vi "camara 3.vi"() -> ()   [LabVIEW 2010]
uses:
  <vilib>/addons/PixeLINK/Low Level Functions/CAMERA_FEATURES.llb/TDPU-CameraFeatures-PixelFormat.ctl
  <vilib>/sound2/lvsound2.llb/Sound Data Format.ctl
  <vilib>/sound2/lvsound2.llb/Sampling Mode.ctl
  <vilib>/Utility/error.llb/DialogType.ctl
  <vilib>/sound2/lvsound2.llb/Sound Output Task ID.ctl
  <vilib>/vision/Image Controls.llb/IMAQ Image.ctl
  <vilib>/addons/PixeLINK/Low Level Functions/ACQUISITION.llb/TDPU-Acquisition-StreamState.ctl
  <vilib>/addons/PixeLINK/Low Level Functions/CAMERA_FEATURES.llb/TDPU-CameraFeatures-FeatureFlags.ctl
  <vilib>/addons/PixeLINK/Low Level Functions/CAMERA_FEATURES.llb/TDPU-CameraFeatures-FeatureIds.ctl
  <vilib>/DAQmx/create/channels.llb/DAQmx Create Channel (AO-Voltage-Basic).vi
  <vilib>/DAQmx/configure/timing.llb/DAQmx Timing (Use Waveform).vi
panel:
  out "time elapsed (ms)":u32
  in  "Calibracion DAQ":T1
  in  "Secuencial":bool=TRUE
  in  "Freq Calibrador":dbl
  in  "Calibrar Sonido":bool
  out "Archivo Actual":path
  out "Guardando Imagen":bool=TRUE
  out "Freq Output":dbl
  out "Saltando":bool=TRUE
  out "Estable":bool=TRUE
  in  "Comienza Saltos":bool=TRUE
  in  "Nombre Imagen":string="foto"
  in  "Path":path
  in  "Parametros de Saltos":T2={"Numero de Saltos"=6, "Paso del Salto (Hz)"=100.0, "Tiempo de estabilizacion (s)"=1.0, "Frequencia de estabilizacion (Hz)"=2000.0, "Tiempo de rampa ON (s)"=5.0, "Tiempo de rampa OFF (s)"=1.0}
  in  "Numero Ultimo Experimento":i32
  in  "Tab Control":enum32{"Camara", "DAQ", "Control", "Sonido"}(tab)
  in  "Pixel Format Requerido":T3 items=["PIXEL_FORMAT_MONO8", "PIXEL_FORMAT_MONO16", "PIXEL_FORMAT_YUV422", "PIXEL_FORMAT_BAYER8_GRBG", "PIXEL_FORMAT_BAYER16_GRBG", "PIXEL_FORMAT_RGB24", "PIXEL_FORMAT_RGB48", "PIXEL_FORMAT_BAYER8_RGGB", "PIXEL_FORMAT_BAYER8_GBRG ", "PIXEL_FORMAT_BAYER8_BGGR ", "PIXEL_FORMAT_BAYER16_RGGB ", "PIXEL_FORMAT_BAYER16_GBRG", "PIXEL_FORMAT_BAYER16_BGGR", "PIXEL_FORMAT_RGB32"]
  in  "Exposure Time (ms)":dbl(slide) scale=0.1..2000.0
  in  "Gain":dbl(slide) scale=0.0..25.0
  in  "Red":sgl(slide) scale=0.0..4.0
  in  "Green":sgl(slide) scale=0.0..4.0
  in  "Blue":sgl(slide) scale=0.0..4.0
  in  "Selector":u16(ring) items=["776002034"]
  out "Numero de Camaras":u32
  in  "Camara ON?":bool
  in  "DAQ Parameters":T4={"Minimum Value"=-10.0, "Maximum Value"=10.0, "Physical Channel"="Dev1/ao0", "DAQ Fs (S/s)"=10000.0}
  in  "Ajuste ON?":bool
  in  "Control ON?":bool
  in  "Reset Control":bool
  in  "lamda (nm)":dbl=546.1
  in  "Control Parameters":T5={"N Init Avg"=6, "N Avg Best"=3, "% Best to test"=0.95, "% Best to beat"=1.0}
  in  "device ID":u32
  in  "sound format":T6={"sample rate (S/s)"=44000.0, "number of channels"=2, "bits per sample"=16}
  in  "Frecuencia":dbl(knob)=2000.0 scale=1000.0..4000.0
  in  "tiempo sonido (ms)":sgl=200.0
  out "Contraste":dbl(graph)
  out "Waveform":waveform(dbl)(graph)
  out "Image":T7(plugin-control)
  in  "Stop App":bool
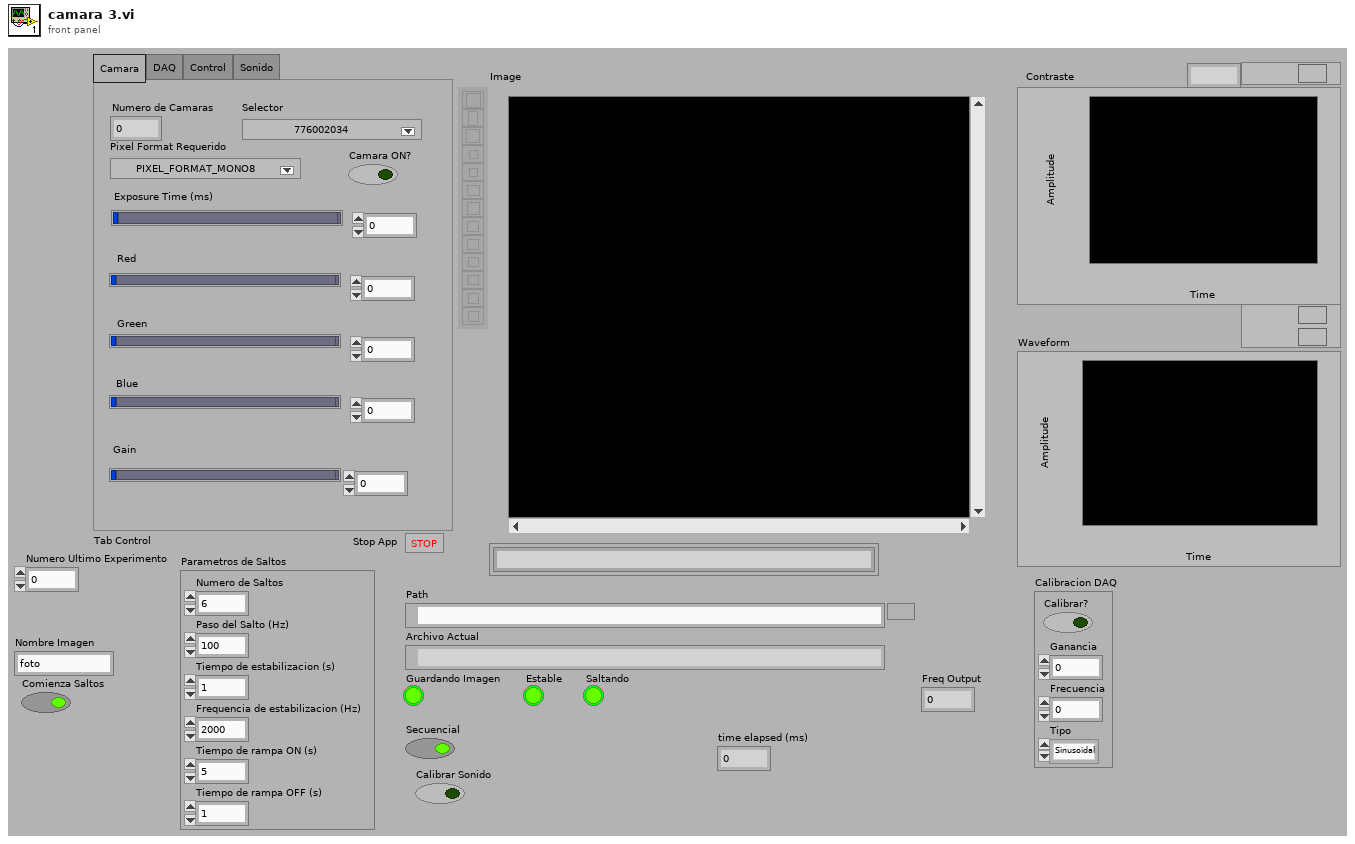
[diagram p1: front panel]
types:
  T1 = cluster{"Calibrar?":bool, "Ganancia":dbl, "Frecuencia":dbl, "Tipo":enum16{"Sinusoidal", "Triangular", "Cuadrada"}}
  T2 = cluster{"Numero de Saltos":i32, "Paso del Salto (Hz)":dbl, "Tiempo de estabilizacion (s)":dbl, "Frequencia de estabilizacion (Hz)":dbl, "Tiempo de rampa ON (s)":dbl, "Tiempo de rampa OFF (s)":dbl}
  T3 = typedef "TDPU-CameraFeatures-PixelFormat.ctl" = u16
  T4 = cluster{"Minimum Value":dbl, "Maximum Value":dbl, "Physical Channel":tag, "DAQ Fs (S/s)":dbl}
  T5 = cluster{"N Init Avg":u32, "N Avg Best":u32, "% Best to test":dbl, "% Best to beat":dbl}
  T6 = typedef "Sound Data Format.ctl" = cluster{"sample rate (S/s)":dbl, "number of channels":i32, "bits per sample":i32}
  T7 = typedef "IMAQ Image.ctl" = refnum<image>
  T8 = cluster{"time (ms)":dbl, "sound format":T6, "device ID":u32}
  T9 = cluster{"hCamera":u32, "Error":errorcluster, "uSerialNumber":u32}
  T10 = typedef "Sound Output Task ID.ctl" = u32
  T11 = cluster{"task ID":T10, "error":errorcluster, "sound format":T6}
  T12 = cluster{"DAQ Fs (S/s)":dbl, "task":refnum<k21>, "error":errorcluster, "Min Value":dbl, "Max Value":dbl}
  T13 = cluster{"Amplitud":dbl, "Media":dbl, "Sigma":dbl}
  T14 = typedef "DialogType.ctl" = u16
  T15 = typedef "Sampling Mode.ctl" = i32
  T16 = typedef "Image Type" = u32
  T17 = cluster{"sample rate (S/s)":dbl, "number of channels":i32, "bits per sample":i32}
  T18 = cluster{"hCamera":u32, "errorCamera":errorcluster}
  T19 = cluster{"hCamera":u32, "Error":errorcluster, "uSerialNumber OUT":u32}
  T20 = typedef "TDPU-Acquisition-StreamState.ctl" = u32
  T21 = typedef "TDPU-CameraFeatures-FeatureIds.ctl" = u32
  T22 = typedef "TDPU-CameraFeatures-FeatureFlags.ctl" = u32
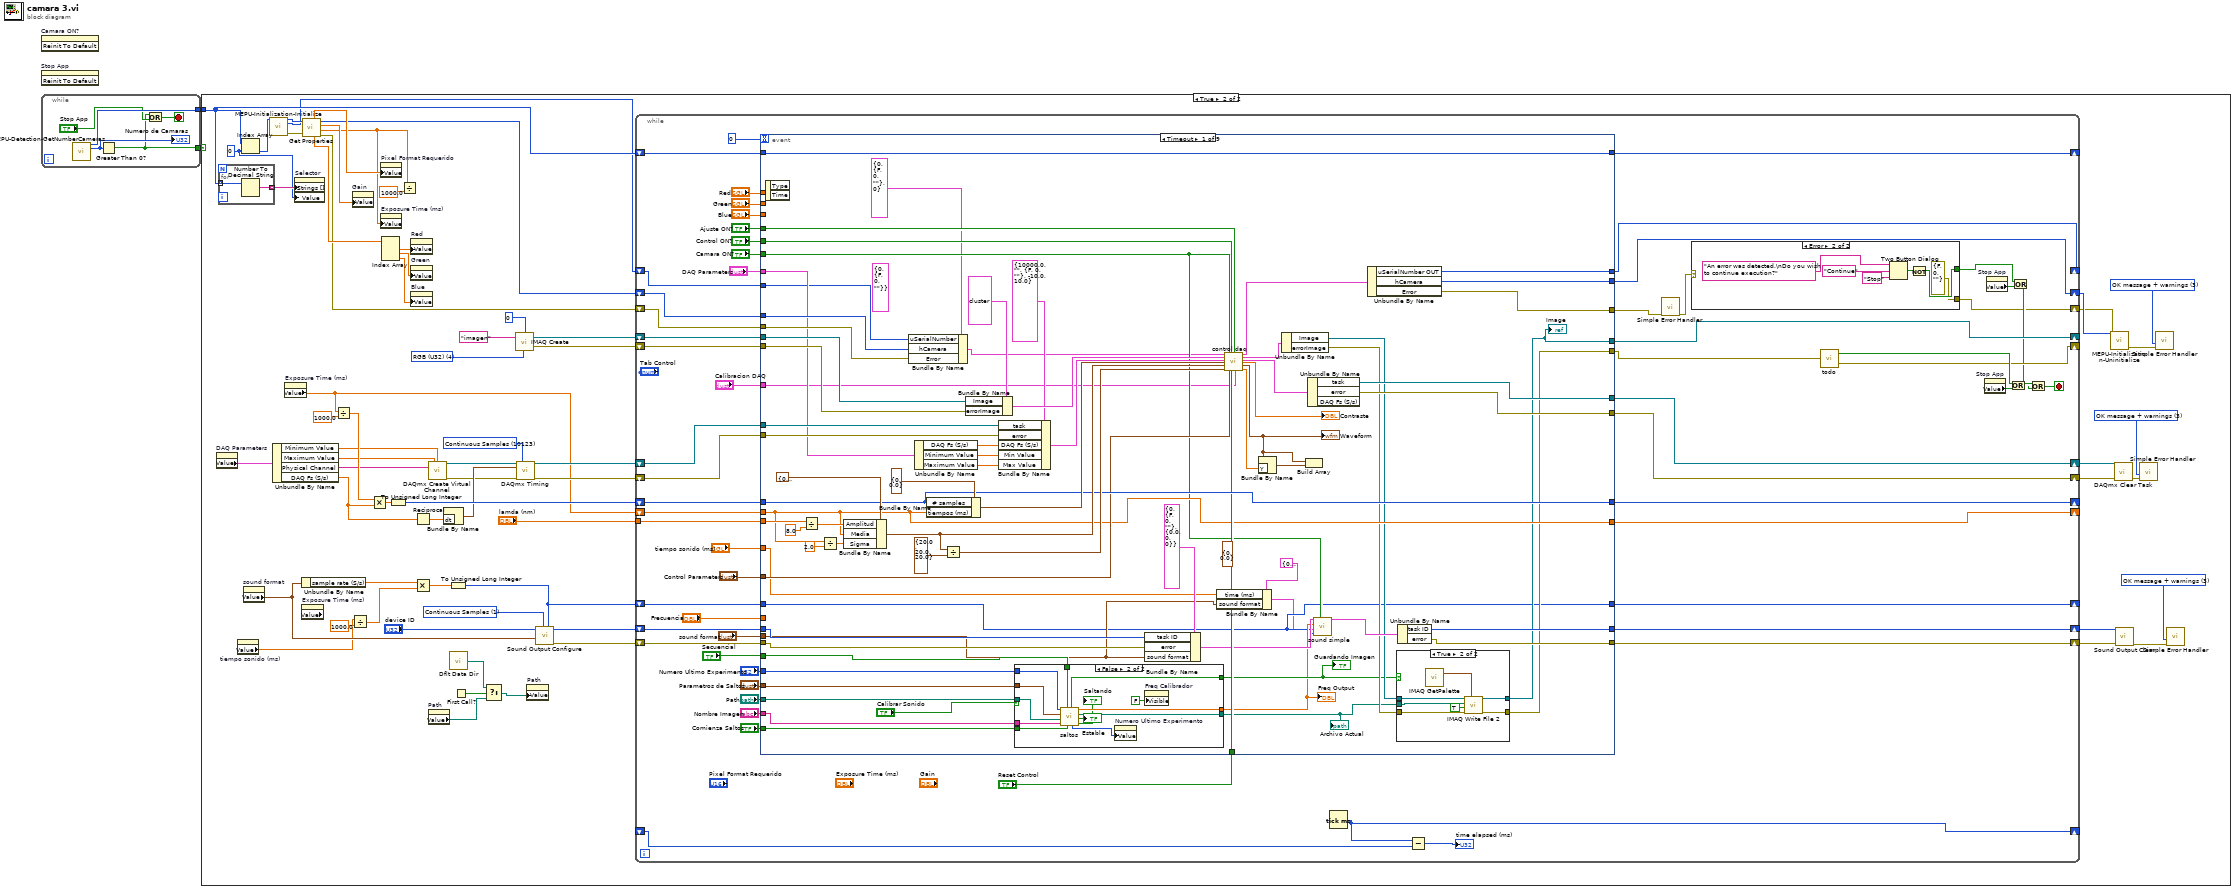
[diagram p0: block diagram]
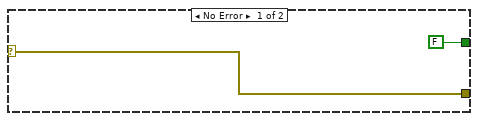
[diagram p3: hidden frame]
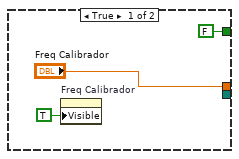
[diagram p4: hidden frame]
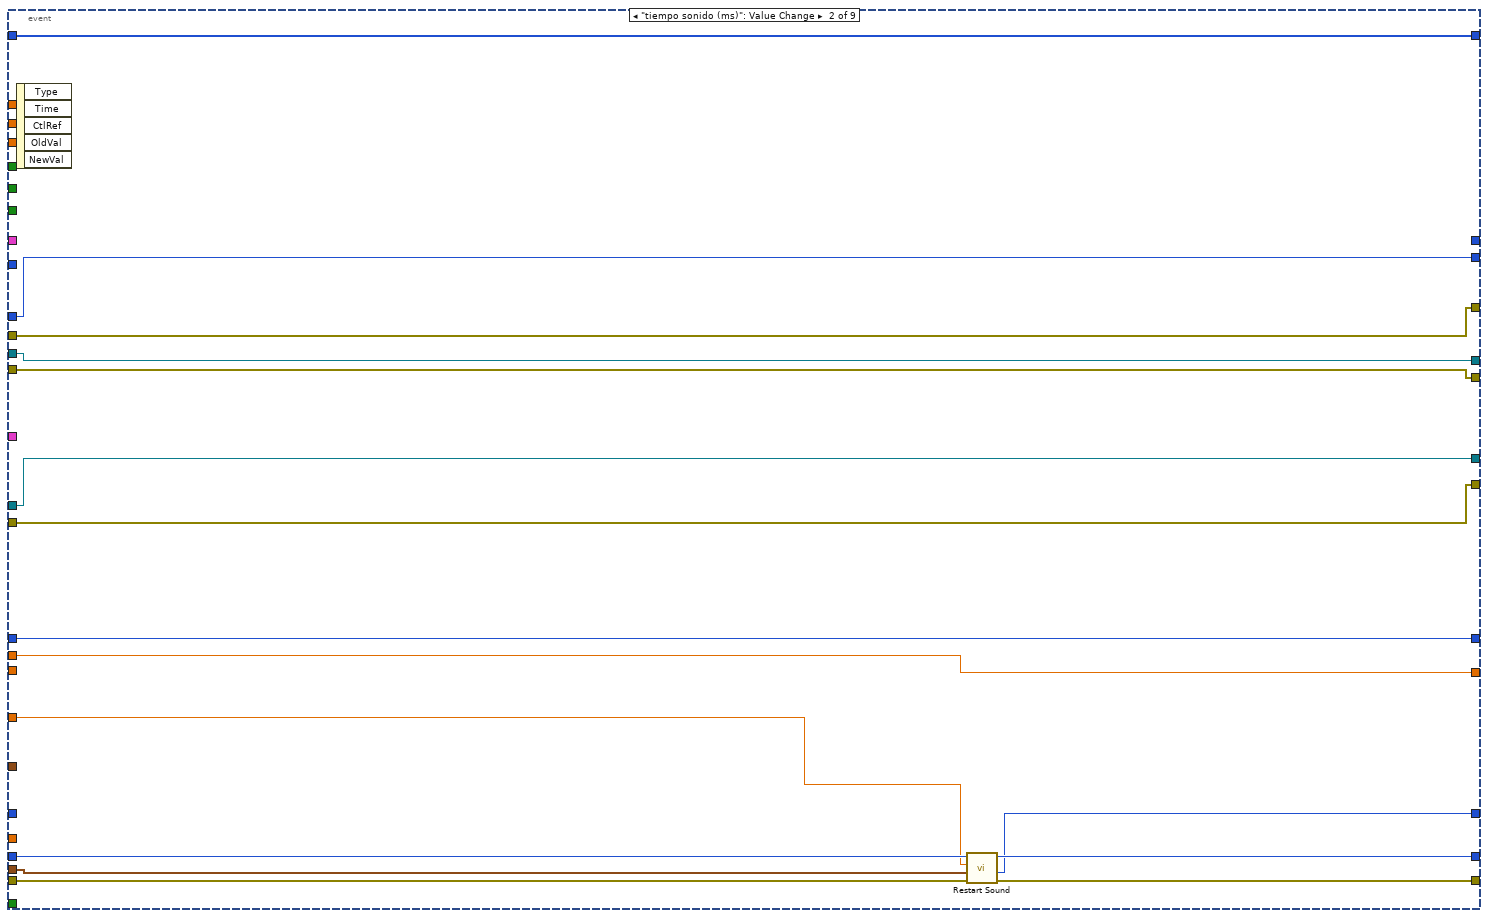
[diagram p6: hidden frame]
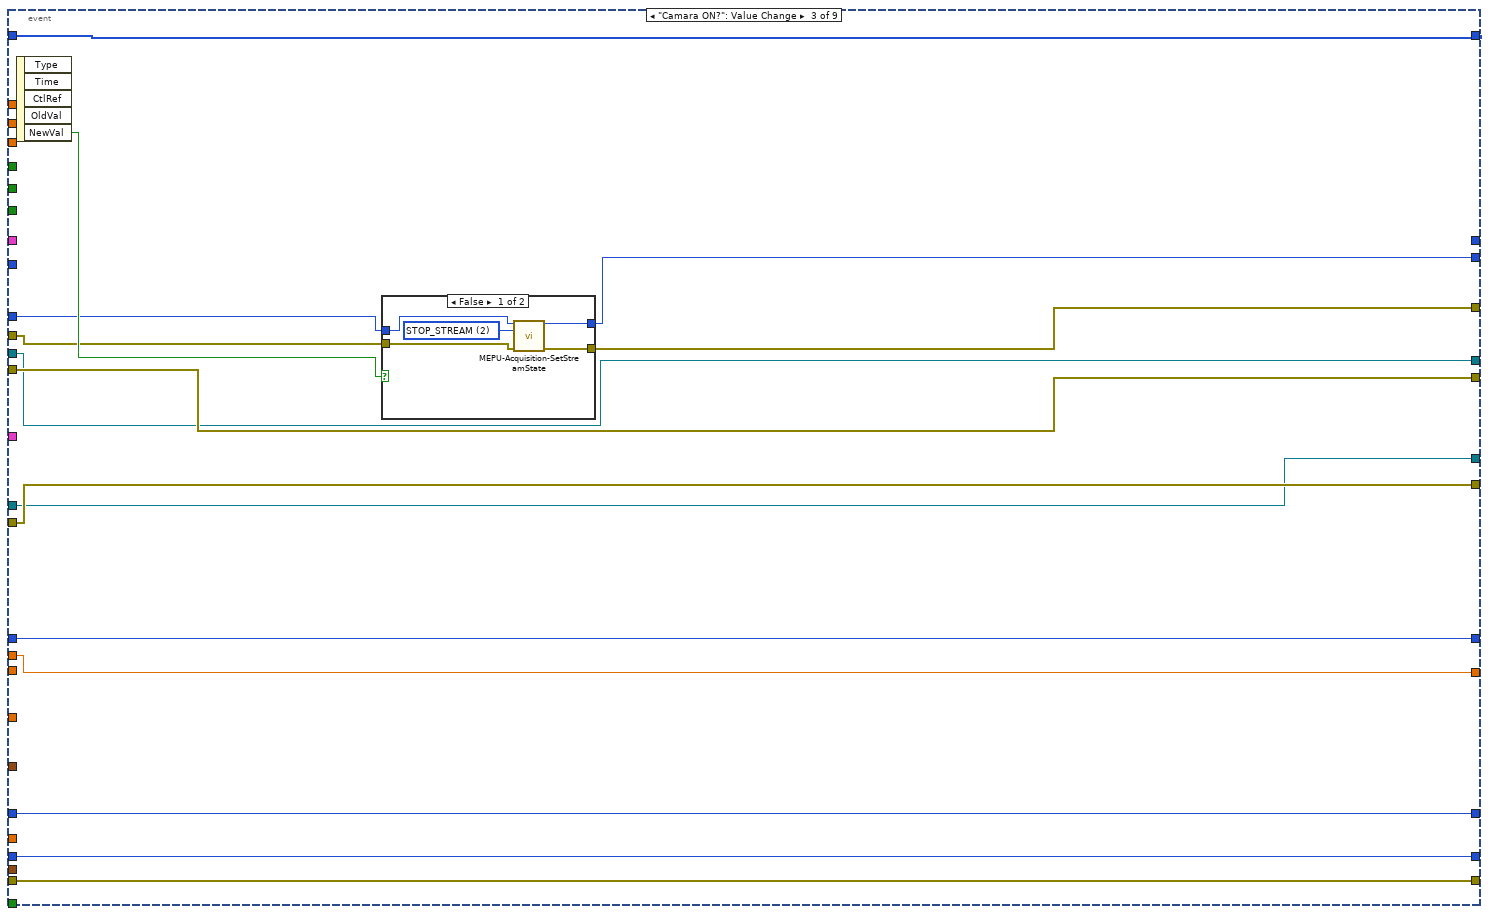
[diagram p7: hidden frame]
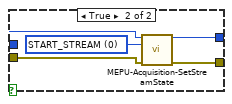
[diagram p8: hidden frame]
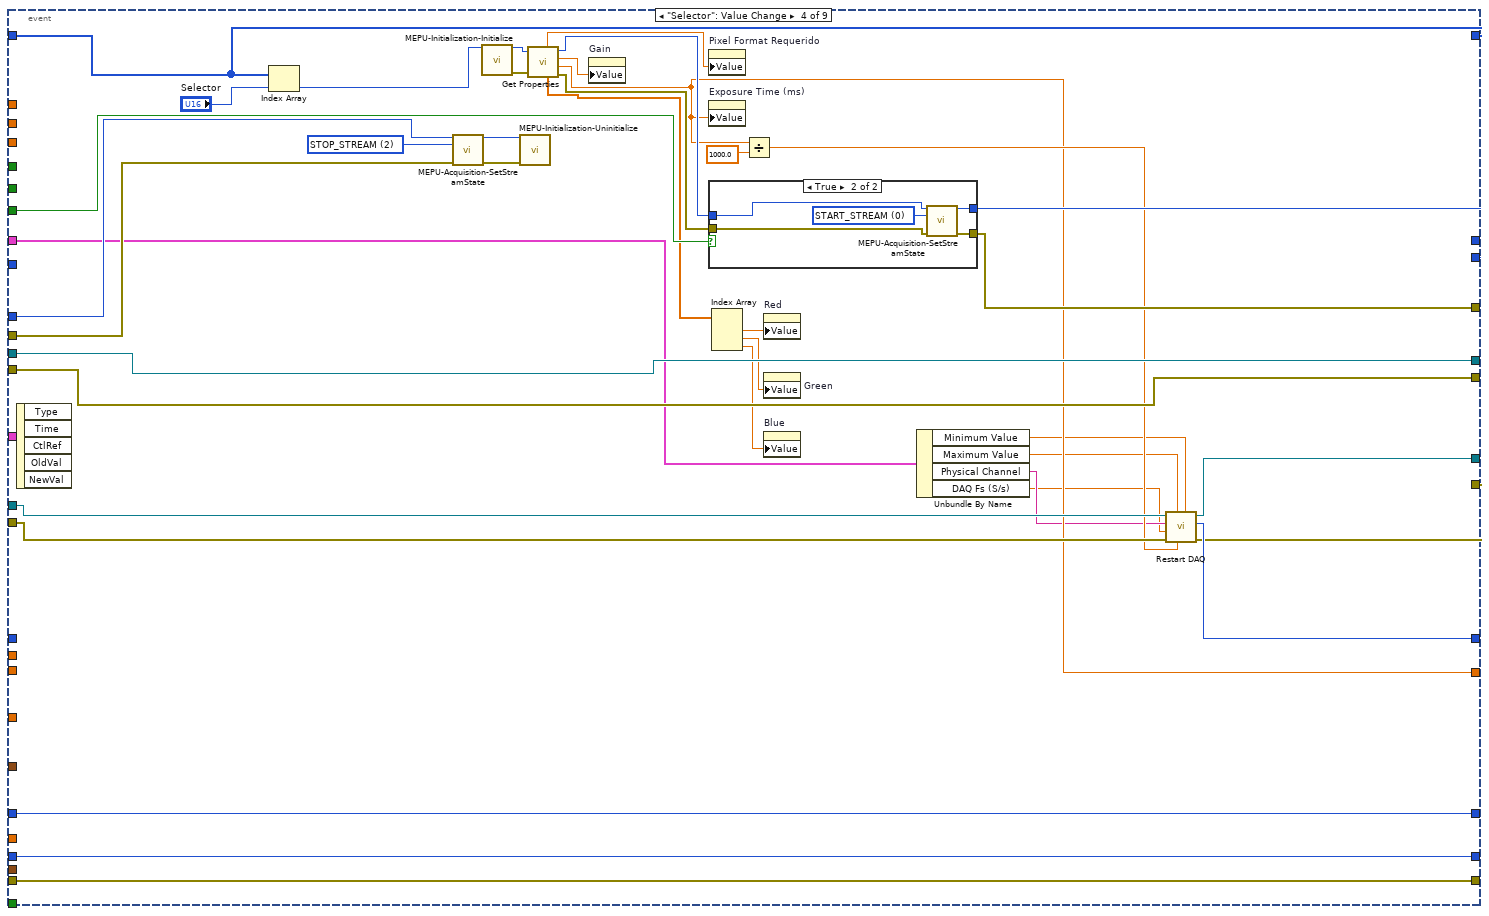
[diagram p9: hidden frame]
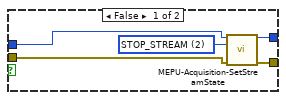
[diagram p10: hidden frame]
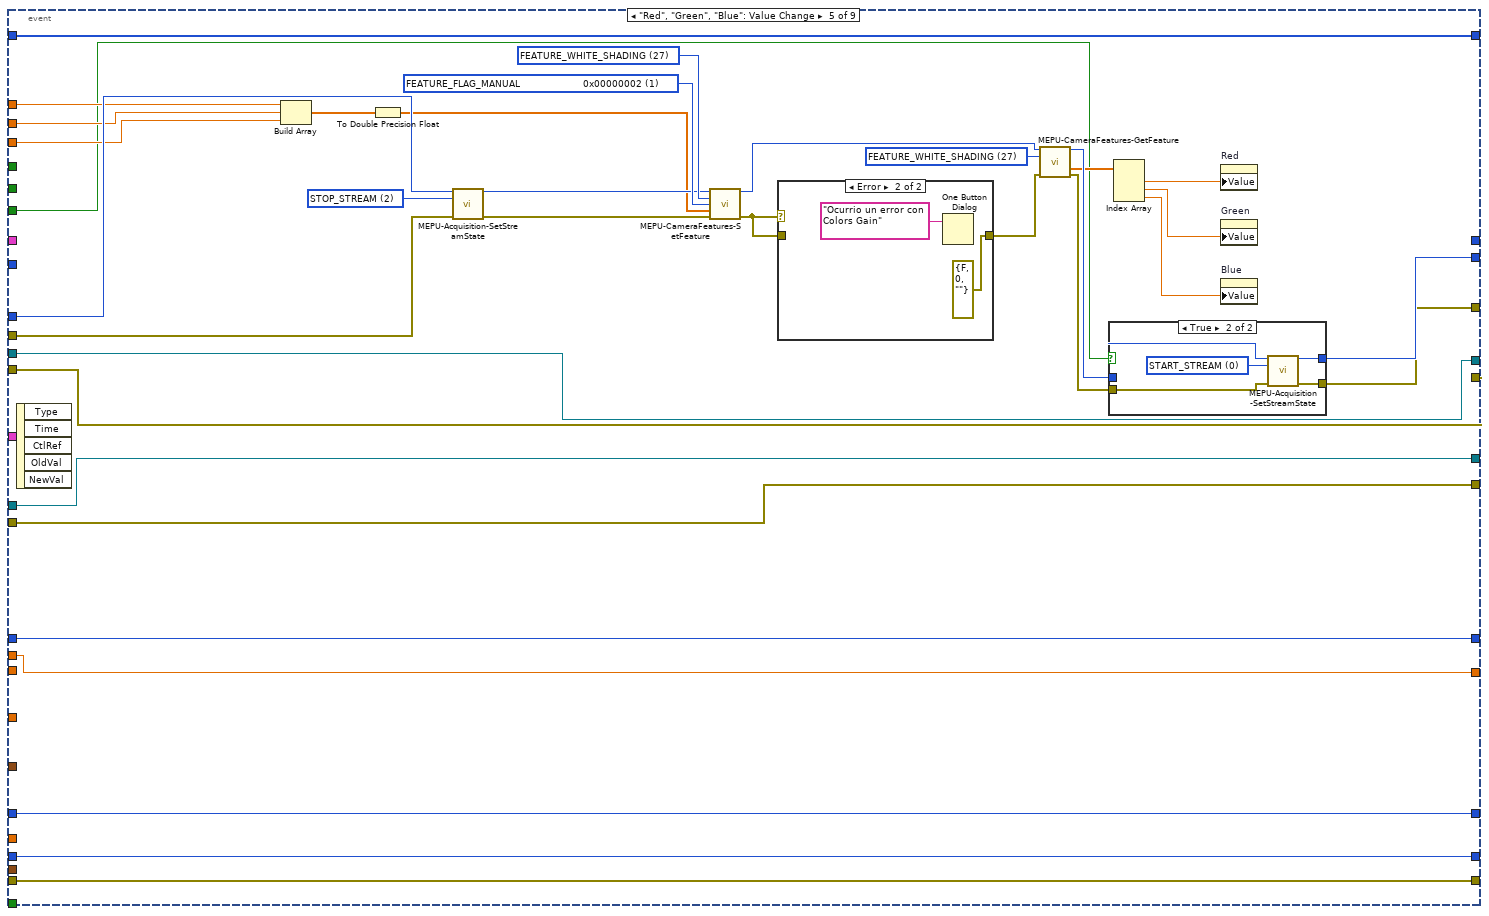
[diagram p11: hidden frame]
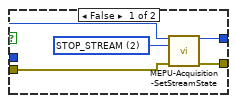
[diagram p12: hidden frame]
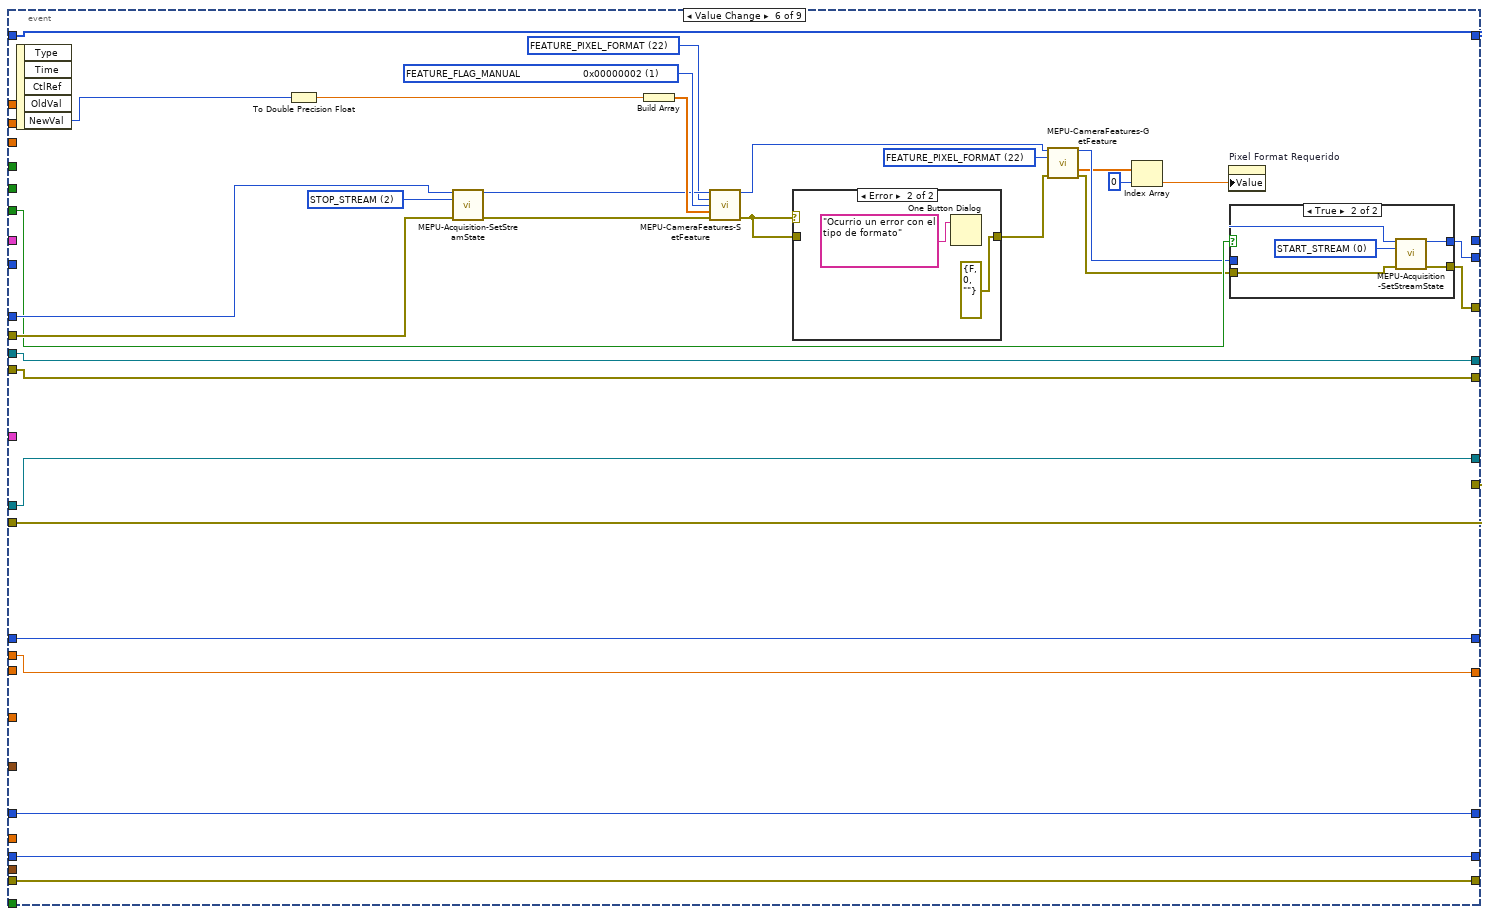
[diagram p14: hidden frame]
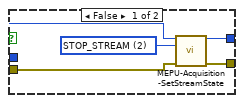
[diagram p15: hidden frame]
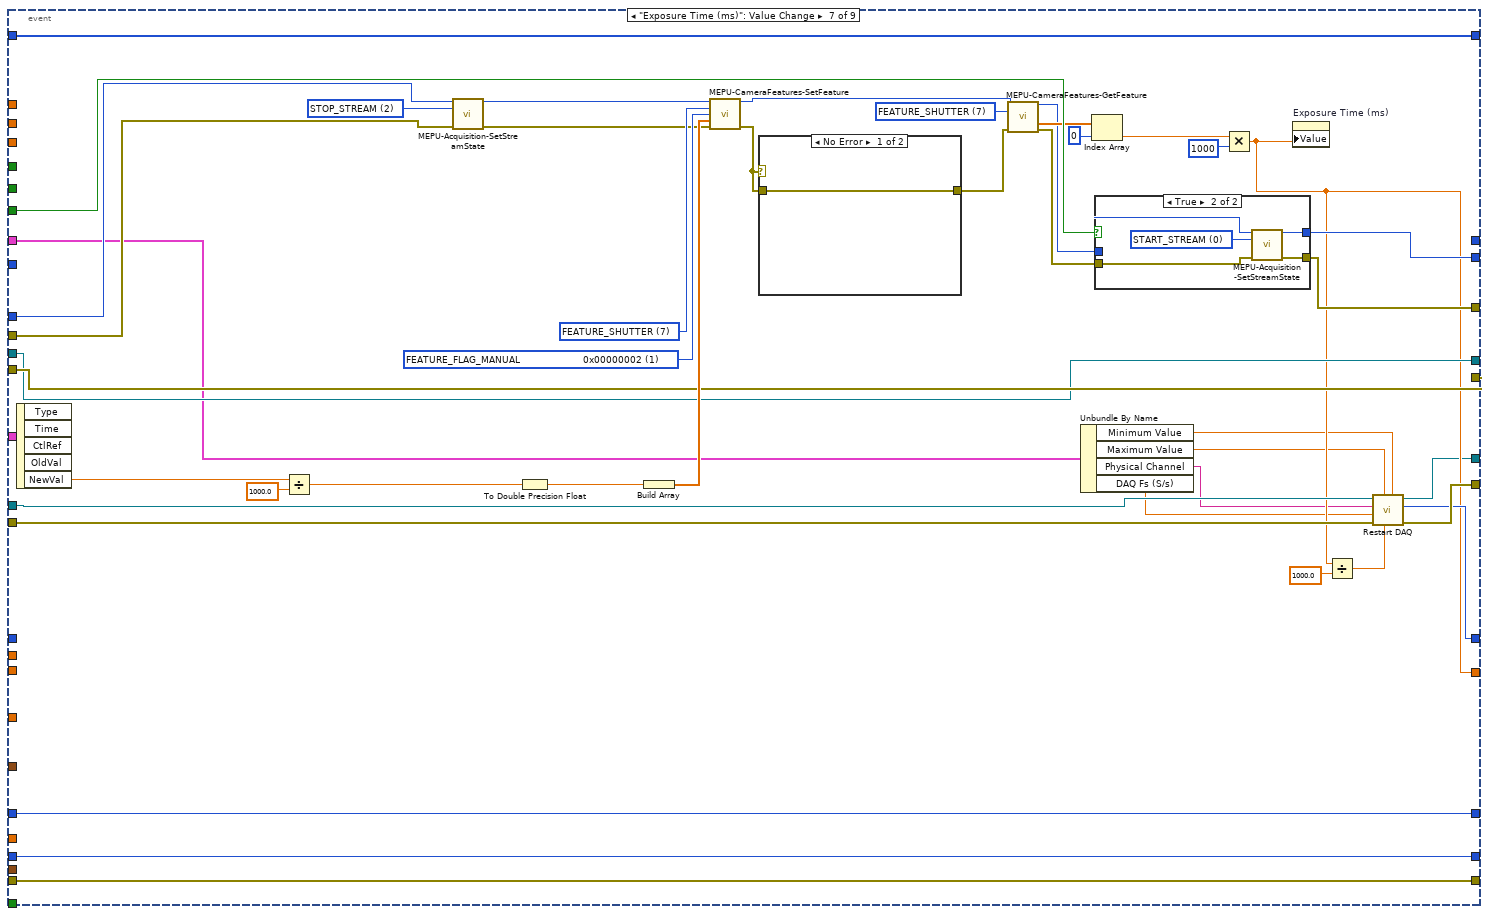
[diagram p17: hidden frame]
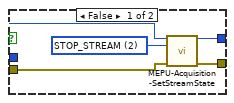
[diagram p18: hidden frame]
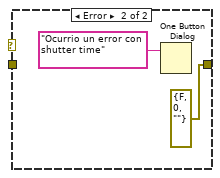
[diagram p19: hidden frame]
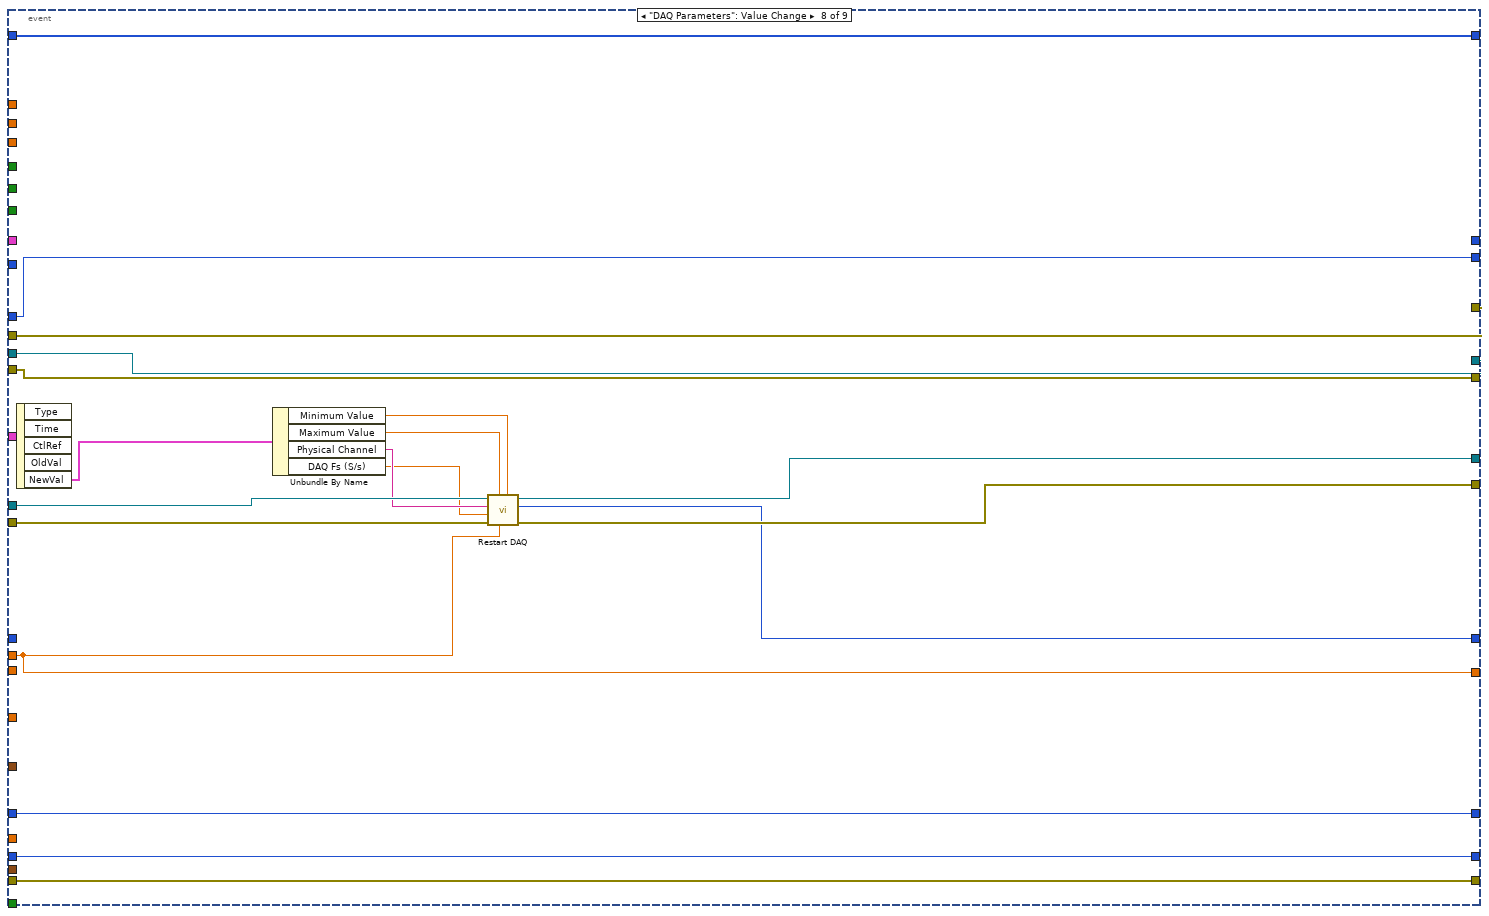
[diagram p20: hidden frame]
diagram:
  n1 = invoke on="Camara ON?" class="Bool (strict)" method="Reinit To Default"() -> ()  [unwired: 3 in, 3 out]
  n2 = invoke on="Stop App" class="Bool (strict)" method="Reinit To Default"() -> ()  [unwired: 3 in, 3 out]
  n3 = while {
    tunnel: [w7] -> w2
    tunnel: [w3] -> w1
    stop <- w5 stop-if-true
    n4 = call <vilib>:"MEPU-Detection-GetNumberCameras.vi"() -> ("LV_SerialNumbers OUT"=w7:u32[], "LV_NumberSerial OUT"=w4:u32)  [unwired: 13 in, 1 out]
    "Numero de Camaras" <- w4
    n5 = Greater Than 0?(x=w4) -> (x > 0?=w3:bool)
    n6 = Or(x=w3, y="Stop App") -> (x .or. y?=w5:bool)
  }
  n7 = case shown="True" w1 {
    tunnel: w2 -> [_ w72]
    frame False {
    }
    frame True {
      w23 = T14 3 items=["no dialog", "OK message", "continue or stop message", "OK message + warnings", "continue/stop + warnings"] ("type of dialog (OK msg:1)")
      w25 = T14 3 items=["no dialog", "OK message", "continue or stop message", "OK message + warnings", "continue/stop + warnings"] ("type of dialog (OK msg:1)")
      w35 = T15 1 items=["Finite Samples", "Continuous Samples"] ("sample mode")
      w38 = T14 3 items=["no dialog", "OK message", "continue or stop message", "OK message + warnings", "continue/stop + warnings"] ("type of dialog (OK msg:1)")
      w47 = 10123 items=["Finite Samples"=10178, "Continuous Samples"=10123, "Hardware Timed Single Point"=12522] ("sample mode")
      w66 = T16 4 items=["Grayscale (U8)", "Grayscale (I16)", "Grayscale (SGL)", "Complex (CSG)", "RGB (U32)", "HSL (U32)", "RGB (U64)", "Grayscale (U16)"] ("Image Type")
      w71 = 0
      n8 = property on="DAQ Parameters" class="Clust (strict)"() -> ("Value"=w16:T4)  [unwired: 2 in, 2 out]
      n9 = for {
        tunnel: w72 -> [w548] mode=indexing
        tunnel: [w547] -> w74 mode=indexing
        n10 = Number To Decimal String(number=w548) -> (decimal integer string=w547:string)  [unwired: 1 in]
      }
      n11 = property on="tiempo sonido (ms)" class="DigNum (strict)"() -> ("Value"=w14:sgl)  [unwired: 2 in, 2 out]
      n12 = Index Array(array=w72, index=w71) -> (element=w73:u32)
      n13 = property on="sound format" class="Clust (strict)"() -> ("Value"=w17:T17)  [unwired: 2 in, 2 out]
      n14 = call <vilib>:"MEPU-Initialization-Initialize.vi"("uSerialNumber IN"=w73) -> ("phCamera OUT"=w65:u32, "uSerialNumber OUT"=w9:u32, "Error OUT"=w64:errorcluster)  [unwired: 12 in]
      n15 = Unbundle By Name(w16) -> ("Minimum Value"=w20:dbl, "Maximum Value"=w19:dbl, "Physical Channel"=w15:tag, "DAQ Fs (S/s)"=w18:dbl)
      n16 = property on="Exposure Time (ms)" class="Slide (strict)"() -> ("Value"=w40:dbl)  [unwired: 2 in, 2 out]
      n17 = property on="Selector" class="Ring (strict)"("Strings []"=w74, "Value"=w71) -> ()  [unwired: 2 in, 2 out]
      n18 = Unbundle By Name(w17) -> ("sample rate (S/s)"=w31:dbl)
      n19 = property on="Exposure Time (ms)" class="Slide (strict)" props=["Value"]() -> ()  [unwired: 2 in, 3 out]
      n20 = call "Get Properties.vi"("hCamera IN"=w65, "Error IN"=w64) -> ("Pixel Format OUT"=w63:dbl, "hCamera OUT"=w49:u32, "Gain OUT"=w62:dbl, "Colors Gain OUT"=w58:dbl[], "Shutter Time OUT (ms)"=w55:dbl, "Error OUT"=w48:errorcluster)  [unwired: 3 in]
      n21 = Divide(x=w40, y=sgl 1000.0) -> (x/y=w51:dbl)
      n22 = Divide(x=w14, y=sgl 1000.0) -> (x/y=w30:sgl)
      n23 = property on="Gain" class="Slide (strict)"("Value"=w62) -> ()  [unwired: 2 in, 2 out]
      n24 = Multiply(x=w51, y=w18) -> (x*y=w57:dbl)
      n25 = property on="Pixel Format Requerido" class="Ring (strict)"("Value"=w63) -> ()  [unwired: 2 in, 2 out]
      n26 = property on="Exposure Time (ms)" class="Slide (strict)"("Value"=w55) -> ()  [unwired: 2 in, 2 out]
      n27 = Index Array(array=w58) -> (element #1=w61:dbl, element #2=w60:dbl, element #3=w59:dbl)  [unwired: 3 in]
      n28 = To Unsigned Long Integer(number=w57) -> (unsigned 32bit integer=w53:u32)
      n29 = Divide(x=w55, y=sgl 1000.0) -> ()  [unwired: 1 out]
      n30 = property on="Red" class="Slide (strict)"("Value"=w61) -> ()  [unwired: 2 in, 2 out]
      n31 = property on="Green" class="Slide (strict)"("Value"=w60) -> ()  [unwired: 2 in, 2 out]
      n32 = property on="Blue" class="Slide (strict)"("Value"=w59) -> ()  [unwired: 2 in, 2 out]
      n33 = Reciprocal(x=w18) -> (1/x=w45:dbl)
      n34 = Multiply(x=w31, y=w30) -> (x*y=w34:dbl)
      n35 = call-poly <vilib>:"DAQmx Create Virtual Channel.vi"("maximum value"=w19, "minimum value"=w20, "physical channels"=w15) -> ("task out"=w44:refnum<k21>, "error out"=w43:errorcluster)  [unwired: 11 in]
      n36 = property on="Path" class="Path"() -> ("Value"=w11:path)  [unwired: 2 in, 2 out]
      n37 = Bundle By Name("dt"=w45) -> (w46:waveform(dbl))  [unwired: 1 in]
      n38 = To Unsigned Long Integer(number=w34) -> (unsigned 32bit integer=w21:u32)
      n39 = call <vilib>:"Dflt Data Dir.vi"() -> ("App:Default Data Directory"=w10:path)
      n40 = First Call?() -> (First Call?: T/F=w13:bool)
      n41 = Select(t=w10, s=w13, f=w11) -> (s? t:f=w12:path)
      n42 = call "IMAQ Create"("Border Size"=0, "Image Name"="imagen", "Image Type"=w66) -> ("New Image"=w69:T7, "error out"=w67:errorcluster)  [unwired: 2 in]
      n43 = call-poly <vilib>:"DAQmx Timing.vi"("task/channels in"=w44, "sample mode"=w47, "waveform"=w46, "error in"=w43) -> ("task out"=w42:refnum<k21>, "error out"=w41:errorcluster)  [unwired: 10 in]
      n44 = property on="Path" class="Path"("Value"=w12) -> ()  [unwired: 2 in, 2 out]
      n45 = call <vilib>:"Sound Output Configure.vi"("number of samples/ch"=w21, "sample mode"=w35, "sound format"=w17, "device ID"="device ID") -> ("error out"=w29:errorcluster, "task ID"=w28:T10)  [unwired: 6 in]
      n46 = while {
        shift-right: [w133] -> _
        shift-left: w72 -> [w134]
        shift-right: [w107] -> w70
        shift-left: w49 -> [w132]
        shift-right: [w106] -> w54
        shift-left: w48 -> [w131]
        shift-right: [w113] -> _
        shift-left: w67 -> [w119]
        shift-right: [w118] -> _
        shift-left: w69 -> [w124]
        shift-right: [w114] -> _
        shift-left: w40 -> [w109]
        tunnel: "lamda (nm)" -> [w108]
        shift-right: [w103] -> _
        shift-left: w53 -> [w112]
        shift-right: [w99] -> w37
        shift-left: w42 -> [w101]
        shift-right: [w98] -> w36
        shift-left: w41 -> [w100]
        shift-right: [w94] -> w27
        shift-left: w28 -> [w96]
        shift-right: [w95] -> w26
        shift-left: w29 -> [w97]
        shift-right: [w92] -> _
        shift-left: w21 -> [w93]
        shift-right: [w79] -> _
        shift-left: w9 -> [w78]
        shift-right: [w76] -> _
        shift-left: _ -> [w77]
        stop <- w121 stop-if-true
        n47 = event shown="[0] Timeout" {
          selector: _ -> [_ _ _ _ _ _ _ _ _]
          dyn-events: _ -> [_ _ _ _ _ _ _ _ _]
          timeout: 0 -> [_ _ _ _ _ _ _ _ _]
          tunnel: w134 -> [w217 w258 w270 w320 w367 w404 w461 w501 w525]
          tunnel: [w196 w246 w268 w313 w351 w403 w460 w497 w524] -> w107
          tunnel: [w195 w247 w267 w314 w350 w402 w459 w498 w523] -> w126
          tunnel: [w217 w258 w270 w320 w367 w404 w461 w501 w525] -> w133
          tunnel: w132 -> [w216 w246 w266 w315 w353 w409 w458 w497 w522]
          tunnel: w131 -> [w215 w247 w265 w316 w352 w408 w457 w498 w521]
          tunnel: "Camara ON?" -> [w154 _ _ w312 w340 w401 w456 _ w520]
          tunnel: w124 -> [w212 w248 w271 w310 w355 w389 w442 w499 w511]
          tunnel: w119 -> [w211 w249 w272 w311 w354 w400 w453 w500 w519]
          tunnel: [w158 w249 w272 w311 w354 w400 w453 w500 w519] -> w123
          tunnel: [w160 w248 w271 w310 w355 w389 w442 w499 w511] -> w118
          tunnel: "Red" -> [_ _ _ _ w345 _ _ _ _]
          tunnel: "Green" -> [_ _ _ _ w344 _ _ _ _]
          tunnel: "Blue" -> [_ _ _ _ w343 _ _ _ _]
          tunnel: [w192 w250 w262 w296 w337 w384 w434 w494 w506] -> w99
          tunnel: [w191 w251 w263 w297 w336 w385 w440 w492 w505] -> w98
          tunnel: w109 -> [w178 w245 w269 _ w339 w387 _ w493 w508]
          tunnel: [w178 w245 w269 w292 w339 w387 w435 w493 w508] -> w114
          tunnel: w112 -> [w189 w252 w264 _ w338 w386 _ _ w507]
          tunnel: w108 -> [w198 _ _ _ _ _ _ _ _]
          tunnel: "Control ON?" -> [w210 _ _ _ _ _ _ _ _]
          tunnel: "Ajuste ON?" -> [w209 _ _ _ _ _ _ _ _]
          tunnel: [w189 w252 w264 w298 w338 w386 w439 w491 w507] -> w103
          tunnel: "Reset Control" -> [w188 _ _ _ _ _ _ _ _]
          tunnel: w101 -> [w186 w250 w262 w295 w337 w384 w438 w496 w506]
          tunnel: w100 -> [w185 w251 w263 w294 w336 w385 w437 w495 w505]
          tunnel: w97 -> [w181 w255 w261 w284 w333 w381 w428 w488 w503]
          tunnel: w96 -> [w182 w254 w260 w285 w334 w382 w426 w489 w502]
          tunnel: [w175 w257 w261 w284 w333 w381 w428 w488 w503] -> w95
          tunnel: [w176 w256 w260 w285 w334 w382 w426 w489 w502] -> w94
          tunnel: w93 -> [w144 _ w259 w286 w335 w383 w427 w490 w504]
          tunnel: "sound format" -> [w145 w243 _ _ _ _ _ _ _]
          tunnel: "Control Parameters" -> [w179 _ _ _ _ _ _ _ _]
          tunnel: "Frecuencia" -> [_ _ _ _ _ _ _ _ _]
          tunnel: [w144 w253 w259 w286 w335 w383 w427 w490 w504] -> w92
          tunnel: "DAQ Parameters" -> [w171 _ _ w291 _ _ w429 _ _]
          tunnel: "tiempo sonido (ms)" -> [w167 w244 _ _ _ _ _ _ _]
          tunnel: "Numero Ultimo Experimento" -> [w166 _ _ _ _ _ _ _ _]
          tunnel: "Parametros de Saltos" -> [w165 _ _ _ _ _ _ _ _]
          tunnel: "Path" -> [w164 _ _ _ _ _ _ _ _]
          tunnel: "Nombre Imagen" -> [w163 _ _ _ _ _ _ _ _]
          tunnel: "Comienza Saltos" -> [w162 _ _ _ _ _ _ _ _]
          tunnel: "Secuencial" -> [w152 _ _ _ _ _ _ _ _]
          tunnel: "Calibracion DAQ" -> [w151 _ _ _ _ _ _ _ _]
          tunnel: w78 -> [w148 _ _ _ _ _ _ _ _]
          tunnel: [w147 _ _ _ _ _ _ _ _] -> w79
          event Timeout {
            (unwired) cluster{"# samples":u32, "tiempos (ms)":dbl} {"# samples"=0, "tiempos (ms)"=0.0} ("Sound Parameters")
            (unwired) T18 {"hCamera"=0, "errorCamera"={"status"=FALSE, "code"=0, "source"=""}} ("Camera Device IN")
            n48 = event-data() -> ()  [unwired: 1 in, 2 out]
            n49 = Divide(x=w198, y=8.0) -> (x/y=w202:dbl)
            n50 = Divide(x=w178, y=2.0) -> (x/y=w205:dbl)
            n51 = Bundle By Name(cluster=T13 {"Amplitud"=0.0, "Media"=0.0, "Sigma"=0.0} ("Parametros Maximos"), "Amplitud"=w202, "Media"=w178, "Sigma"=w205) -> (w200:T13)
            n52 = Bundle By Name(cluster=T9 {"hCamera"=0, "Error"={"status"=FALSE, "code"=0, "source"=""}, "uSerialNumber"=0} ("Camera Device  IN"), "uSerialNumber"=w148, "hCamera"=w216, "Error"=w215) -> (w149:T9)
            n53 = Unbundle By Name(w171) -> ("DAQ Fs (S/s)"=w174:dbl, "Minimum Value"=w173:dbl, "Maximum Value"=w172:dbl)
            n54 = Bundle By Name(cluster=cluster{"# samples":u32, "tiempos (ms)":dbl} {"# samples"=0, "tiempos (ms)"=0.0} ("Sound Parameters"), "# samples"=w189, "tiempos (ms)"=w178) -> (w207:cluster{"# samples":u32, "tiempos (ms)":dbl})
            n55 = Divide(x=w200, y=T13 {"Amplitud"=20.0, "Media"=20.0, "Sigma"=20.0}) -> (x/y=w199:T13)
            n56 = Bundle By Name(cluster=cluster{"Image":T7, "errorImage":errorcluster} {"Image"=refnum, "errorImage"={"status"=FALSE, "code"=0, "source"=""}} ("Image Device IN"), "Image"=w212, "errorImage"=w211) -> (w213:cluster{"Image":T7, "errorImage":errorcluster})
            n57 = Bundle By Name(cluster=T12 {"DAQ Fs (S/s)"=10000.0, "task"="", "error"={"status"=FALSE, "code"=0, "source"=""}, "Min Value"=-10.0, "Max Value"=10.0} ("DAQ Device"), "task"=w186, "error"=w185, "DAQ Fs (S/s)"=w174, "Min Value"=w173, "Max Value"=w172) -> (w187:T12)
            n58 = case shown="False" "Calibrar Sonido" {
              tunnel: w166 -> [_ w233]
              tunnel: w165 -> [_ w232]
              tunnel: w164 -> [_ w231]
              tunnel: w163 -> [_ w230]
              tunnel: w162 -> [_ w229]
              tunnel: [_ w228] -> w157
              tunnel: [FALSE ("Captura Imagen") w227] -> w156
              tunnel: ["Freq Calibrador" w226] -> w155
              tunnel: w152 -> [_ w221]
              frame True {
                n59 = property on="Freq Calibrador" class="DigNum (strict)"("Visible"=TRUE) -> ()  [unwired: 2 in, 2 out]
              }
              frame False {
                n60 = call "saltos.vi"("Comienza Saltos"=w229, "Secuencial"=w221, "Nombre Imagen"=w230, "Path"=w231, "Parametros de Saltos"=w232, "Numero Ultimo Experimento"=w233) -> ("Tomando Saltos"=→"Saltando":bool, "Estable"=→"Estable":bool, "appended path"=w228:path, "Freq Output"=w226:dbl, "Numero Actual Experimento"=w225:i32, "Captura Imagen"=w227:bool)
                n61 = property on="Numero Ultimo Experimento" class="DigNum (strict)"("Value"=w225) -> ()  [unwired: 2 in, 2 out]
                n62 = property on="Freq Calibrador" class="DigNum (strict)"("Visible"=FALSE) -> ()  [unwired: 2 in, 2 out]
              }
            }
            "Freq Output" <- w155
            "Guardando Imagen" <- w156
            "Archivo Actual" <- w157
            n63 = Bundle By Name(cluster=T11 {"task ID"=0, "error"={"status"=FALSE, "code"=0, "source"=""}, "sound format"={"sample rate (S/s)"=0.0, "number of channels"=0, "bits per sample"=0}} ("Sound Device IN"), "task ID"=w182, "error"=w181, "sound format"=w145) -> (w180:T11)
            n64 = Bundle By Name(cluster=T8 {"time (ms)"=0.0, "sound format"={"sample rate (S/s)"=0.0, "number of channels"=0, "bits per sample"=0}, "device ID"=0} ("Sound Parameters"), "time (ms)"=w167, "sound format"=w145) -> (w143:T8)
            n65 = call "control daq.vi"("Camera Device  IN"=w149, "Image Device IN"=w213, "DAQ Device IN"=w187, "Time Control Parameters"=w207, "Parametros Maximos"=w200, "detla Parametros"=w199, "Camara ON?"=w154, "Control Parameters"=w179, "Control?"=w210, "Reset Control"=w188, "Ajuste?"=w209, "Calibracion DAQ"=w151) -> ("Camera Device OUT"=w197:T19, "Image Device OUT"=w194:cluster{"Image":T7, "errorImage":errorcluster}, "DAQ Device OUT"=w193:T12, "Contraste"=→"Contraste":dbl, "Waveform"=w168:waveform(dbl), "Señal de Control"=w170:dbl[])  [unwired: 2 in]
            "Waveform" <- w168
            n66 = Bundle By Name(cluster=w168, "Y"=w170) -> (w169:waveform(dbl))
            n67 = Unbundle By Name(w194) -> ("Image"=w161:T7, "errorImage"=w159:errorcluster)
            n68 = Build Array(w168, w169) -> ()  [unwired: 1 out]
            n69 = Unbundle By Name(w193) -> ("task"=w192:refnum<k21>, "error"=w191:errorcluster)  [unwired: 1 out]
            n70 = call "sound simple.vi"("sound?"=w154, "# samples"=w144, "Sound Parameters"=w143, "Frecuencia"=w155, "Sound Device IN"=w180) -> ("Sound Device OUT"=w177:T11)  [unwired: 3 in, 1 out]
            n71 = Unbundle By Name(w197) -> ("uSerialNumber OUT"=w147:u32, "hCamera"=w196:u32, "Error"=w195:errorcluster)
            n72 = case shown="True" w156 {
              tunnel: w161 -> [w235 w242]
              tunnel: [w235 w241] -> w160
              tunnel: w159 -> [w234 w240]
              tunnel: [w234 w239] -> w158
              tunnel: w157 -> [_ w238]
              frame False {
              }
              frame True {
                n73 = call "IMAQ GetPalette"() -> ("Color Palette"=w237:cluster{"Red":u8, "Green":u8, "Blue":u8}[])  [unwired: 5 in, 1 out]
                n74 = call-poly "IMAQ Write File 2"("Color Palette"=w237, "error in (no error)"=w240, "Compress? (N)"=TRUE, "File Path"=w238, "Image"=w242) -> ("error out"=w239:errorcluster, "Image Out (duplicate)"=w241:T7)  [unwired: 5 in]
              }
            }
            "Image" <- w160
            n75 = Unbundle By Name(w177) -> ("task ID"=w176:T10, "error"=w175:errorcluster)
          }
          event "tiempo sonido (ms)": Value Change {
            n76 = event-data() -> ()  [unwired: 1 in, 5 out]
            n77 = call "Restart Sound.vi"("error IN"=w255, "sound format"=w243, "time (ms)"=w244, "task ID IN"=w254) -> ("error OUT"=w257:errorcluster, "# samples"=w253:u32, "task ID OUT"=w256:T10)  [unwired: 1 in]
          }
          event "Camara ON?": Value Change {
            n78 = event-data() -> ("NewVal"=w273:bool)  [unwired: 1 in, 4 out]
            n79 = case shown="False" w273 {
              tunnel: w266 -> [w274 w282]
              tunnel: w265 -> [w277 w281]
              tunnel: [w275 w280] -> w267
              tunnel: [w276 w279] -> w268
              frame False {
                w278 = T20 2 items=["START_STREAM", "PAUSE_STREAM", "STOP_STREAM"] ("uStreamState IN")
                n80 = call <vilib>:"MEPU-Acquisition-SetStreamState.vi"("hCamera IN"=w274, "uStreamState IN"=w278, "Error IN"=w277) -> ("hCamera OUT"=w276:u32, "Error OUT"=w275:errorcluster)  [unwired: 11 in]
              }
              frame True {
                w283 = T20 0 items=["START_STREAM", "PAUSE_STREAM", "STOP_STREAM"] ("uStreamState IN")
                n81 = call <vilib>:"MEPU-Acquisition-SetStreamState.vi"("hCamera IN"=w282, "uStreamState IN"=w283, "Error IN"=w281) -> ("hCamera OUT"=w279:u32, "Error OUT"=w280:errorcluster)  [unwired: 11 in]
              }
            }
          }
          event "Selector": Value Change {
            w319 = T20 2 items=["START_STREAM", "PAUSE_STREAM", "STOP_STREAM"] ("uStreamState IN")
            n82 = event-data() -> ()  [unwired: 1 in, 5 out]
            n83 = Index Array(array=w320, index="Selector") -> (element=w321:u32)
            n84 = call <vilib>:"MEPU-Acquisition-SetStreamState.vi"("hCamera IN"=w315, "uStreamState IN"=w319, "Error IN"=w316) -> ("hCamera OUT"=w317:u32, "Error OUT"=w318:errorcluster)  [unwired: 11 in]
            n85 = call <vilib>:"MEPU-Initialization-Initialize.vi"("uSerialNumber IN"=w321) -> ("phCamera OUT"=w306:u32, "Error OUT"=w305:errorcluster)  [unwired: 12 in, 1 out]
            n86 = call <vilib>:"MEPU-Initialization-Uninitialize.vi"("hCamera IN"=w317, "Error IN"=w318) -> ()  [unwired: 13 in, 1 out]
            n87 = call "Get Properties.vi"("hCamera IN"=w306, "Error IN"=w305) -> ("Pixel Format OUT"=w304:dbl, "hCamera OUT"=w302:u32, "Gain OUT"=w301:dbl, "Colors Gain OUT"=w300:dbl[], "Shutter Time OUT (ms)"=w292:dbl, "Error OUT"=w303:errorcluster)  [unwired: 3 in]
            n88 = property on="Gain" class="Slide (strict)"("Value"=w301) -> ()  [unwired: 2 in, 2 out]
            n89 = property on="Pixel Format Requerido" class="Ring (strict)"("Value"=w304) -> ()  [unwired: 2 in, 2 out]
            n90 = property on="Exposure Time (ms)" class="Slide (strict)"("Value"=w292) -> ()  [unwired: 2 in, 2 out]
            n91 = case shown="True" w312 {
              tunnel: [w325 w331] -> w314
              tunnel: [w326 w330] -> w313
              tunnel: w303 -> [w324 w329]
              tunnel: w302 -> [w323 w328]
              frame False {
                w327 = T20 2 items=["START_STREAM", "PAUSE_STREAM", "STOP_STREAM"] ("uStreamState IN")
                n92 = call <vilib>:"MEPU-Acquisition-SetStreamState.vi"("hCamera IN"=w323, "uStreamState IN"=w327, "Error IN"=w324) -> ("hCamera OUT"=w326:u32, "Error OUT"=w325:errorcluster)  [unwired: 11 in]
              }
              frame True {
                w332 = T20 0 items=["START_STREAM", "PAUSE_STREAM", "STOP_STREAM"] ("uStreamState IN")
                n93 = call <vilib>:"MEPU-Acquisition-SetStreamState.vi"("hCamera IN"=w328, "uStreamState IN"=w332, "Error IN"=w329) -> ("hCamera OUT"=w330:u32, "Error OUT"=w331:errorcluster)  [unwired: 11 in]
              }
            }
            n94 = Index Array(array=w300) -> (element #1=w309:dbl, element #2=w308:dbl, element #3=w307:dbl)  [unwired: 3 in]
            n95 = Divide(x=w292, y=sgl 1000.0) -> (x/y=w293:dbl)
            n96 = property on="Red" class="Slide (strict)"("Value"=w309) -> ()  [unwired: 2 in, 2 out]
            n97 = property on="Green" class="Slide (strict)"("Value"=w308) -> ()  [unwired: 2 in, 2 out]
            n98 = property on="Blue" class="Slide (strict)"("Value"=w307) -> ()  [unwired: 2 in, 2 out]
            n99 = Unbundle By Name(w291) -> ("Minimum Value"=w290:dbl, "Maximum Value"=w289:dbl, "Physical Channel"=w288:tag, "DAQ Fs (S/s)"=w287:dbl)
            n100 = call "Restart DAQ.vi"("Min Value"=w290, "tiempo (s)"=w293, "Max Value"=w289, "error IN"=w294, "Fs (S/s)"=w287, "Physical Channel"=w288, "task IN"=w295) -> ("error OUT"=w297:errorcluster, "# samples"=w298:u32, "task OUT"=w296:refnum<k21>)  [unwired: 2 in]
          }
          event "Red", "Green", "Blue": Value Change {
            w360 = T21 27 items=["FEATURE_BRIGHTNESS", "FEATURE_EXPOSURE", "FEATURE_SHARPNESS", "FEATURE_WHITE_BAL", "FEATURE_HUE", "FEATURE_SATURATION", "FEATURE_GAMMA", "FEATURE_SHUTTER", "FEATURE_GAIN", "FEATURE_IRIS", "FEATURE_FOCUS", "FEATURE_TEMPERATURE", "FEATURE_TRIGGER", "FEATURE_ZOOM", "FEATURE_PAN", "FEATURE_TILT", "FEATURE_OPT_FILTER", "FEATURE_GPIO", "FEATURE_FRAME_RATE", "FEATURE_ROI", "FEATURE_FLIP", "FEATURE_PIXEL_ADDRESSING", "FEATURE_PIXEL_FORMAT", "FEATURE_EXTENDED_SHUTTER", "FEATURE_AUTO_ROI", "FEATURE_LOOKUP_TABLE", "FEATURE_MEMORY_CHANNEL", "FEATURE_WHITE_SHADING", "FEATURE_ROTATE", "FEATURE_IMAGER_CLK_DIVISOR", "FEATURE_TRIG_WITH_CNTRLD_LIGHT", "FEATURE_MAX_PIXEL_SIZE"] ("uFeatureId IN")
            w361 = T20 2 items=["START_STREAM", "PAUSE_STREAM", "STOP_STREAM"] ("uStreamState IN")
            w365 = T22 1 items=["FEATURE_FLAG_PRESENCE                 0x00000001", "FEATURE_FLAG_MANUAL                     0x00000002", "FEATURE_FLAG_AUTO                         0x00000004", "FEATURE_FLAG_ONEPUSH                   0x00000008", "FEATURE_FLAG_OFF                            0x00000010", "FEATURE_FLAG_DESC_SUPPORTED    0x00000020", "FEATURE_FLAG_READ_ONLY               0x00000040"] ("uFlags IN")
            w366 = T21 27 items=["FEATURE_BRIGHTNESS", "FEATURE_EXPOSURE", "FEATURE_SHARPNESS", "FEATURE_WHITE_BAL", "FEATURE_HUE", "FEATURE_SATURATION", "FEATURE_GAMMA", "FEATURE_SHUTTER", "FEATURE_GAIN", "FEATURE_IRIS", "FEATURE_FOCUS", "FEATURE_TEMPERATURE", "FEATURE_TRIGGER", "FEATURE_ZOOM", "FEATURE_PAN", "FEATURE_TILT", "FEATURE_OPT_FILTER", "FEATURE_GPIO", "FEATURE_FRAME_RATE", "FEATURE_ROI", "FEATURE_FLIP", "FEATURE_PIXEL_ADDRESSING", "FEATURE_PIXEL_FORMAT", "FEATURE_EXTENDED_SHUTTER", "FEATURE_AUTO_ROI", "FEATURE_LOOKUP_TABLE", "FEATURE_MEMORY_CHANNEL", "FEATURE_WHITE_SHADING", "FEATURE_ROTATE", "FEATURE_IMAGER_CLK_DIVISOR", "FEATURE_TRIG_WITH_CNTRLD_LIGHT", "FEATURE_MAX_PIXEL_SIZE"] ("uFeatureId IN")
            n101 = event-data() -> ()  [unwired: 1 in, 5 out]
            n102 = Build Array(w345, w344, w343) -> (w342:sgl[])
            n103 = To Double Precision Float(number=w342) -> (double precision float=w341:dbl[])
            n104 = call <vilib>:"MEPU-Acquisition-SetStreamState.vi"("hCamera IN"=w353, "uStreamState IN"=w361, "Error IN"=w352) -> ("hCamera OUT"=w363:u32, "Error OUT"=w362:errorcluster)  [unwired: 11 in]
            n105 = call <vilib>:"MEPU-CameraFeatures-SetFeature.vi"("hCamera IN"=w363, "uFeatureId IN"=w366, "uFlags IN"=w365, "pParms IN"=w341, "Error IN"=w362) -> ("hCamera OUT"=w359:u32, "Error OUT"=w364:errorcluster)  [unwired: 8 in, 1 out]
            n106 = case shown="Error" w364 {
              tunnel: [w378 errorcluster {"status"=FALSE, "code"=0, "source"=""} ("Error OUT")] -> w356
              tunnel: w364 -> [w378 _]
              frame No Error {
              }
              frame Error {
                n107 = One Button Dialog(message="Ocurrio un error con Colors Gain") -> ()  [unwired: 1 in, 1 out]
              }
            }
            n108 = call <vilib>:"MEPU-CameraFeatures-GetFeature.vi"("hCamera IN"=w359, "uFeatureId IN"=w360, "Error IN"=w356) -> ("hCamera OUT"=w358:u32, "pParms OUT"=w346:dbl[], "Error OUT"=w357:errorcluster)  [unwired: 8 in, 2 out]
            n109 = case shown="True" w340 {
              tunnel: w357 -> [w371 w376]
              tunnel: [w369 w375] -> w350
              tunnel: [w370 w374] -> w351
              tunnel: w358 -> [w368 w373]
              frame False {
                w372 = T20 2 items=["START_STREAM", "PAUSE_STREAM", "STOP_STREAM"] ("uStreamState IN")
                n110 = call <vilib>:"MEPU-Acquisition-SetStreamState.vi"("hCamera IN"=w368, "uStreamState IN"=w372, "Error IN"=w371) -> ("hCamera OUT"=w370:u32, "Error OUT"=w369:errorcluster)  [unwired: 11 in]
              }
              frame True {
                w377 = T20 0 items=["START_STREAM", "PAUSE_STREAM", "STOP_STREAM"] ("uStreamState IN")
                n111 = call <vilib>:"MEPU-Acquisition-SetStreamState.vi"("hCamera IN"=w373, "uStreamState IN"=w377, "Error IN"=w376) -> ("hCamera OUT"=w374:u32, "Error OUT"=w375:errorcluster)  [unwired: 11 in]
              }
            }
            n112 = Index Array(array=w346) -> (element #1=w349:dbl, element #2=w348:dbl, element #3=w347:dbl)  [unwired: 3 in]
            n113 = property on="Red" class="Slide (strict)"("Value"=w349) -> ()  [unwired: 2 in, 2 out]
            n114 = property on="Green" class="Slide (strict)"("Value"=w348) -> ()  [unwired: 2 in, 2 out]
            n115 = property on="Blue" class="Slide (strict)"("Value"=w347) -> ()  [unwired: 2 in, 2 out]
          }
          event Value Change {
            w394 = T21 22 items=["FEATURE_BRIGHTNESS", "FEATURE_EXPOSURE", "FEATURE_SHARPNESS", "FEATURE_WHITE_BAL", "FEATURE_HUE", "FEATURE_SATURATION", "FEATURE_GAMMA", "FEATURE_SHUTTER", "FEATURE_GAIN", "FEATURE_IRIS", "FEATURE_FOCUS", "FEATURE_TEMPERATURE", "FEATURE_TRIGGER", "FEATURE_ZOOM", "FEATURE_PAN", "FEATURE_TILT", "FEATURE_OPT_FILTER", "FEATURE_GPIO", "FEATURE_FRAME_RATE", "FEATURE_ROI", "FEATURE_FLIP", "FEATURE_PIXEL_ADDRESSING", "FEATURE_PIXEL_FORMAT", "FEATURE_EXTENDED_SHUTTER", "FEATURE_AUTO_ROI", "FEATURE_LOOKUP_TABLE", "FEATURE_MEMORY_CHANNEL", "FEATURE_WHITE_SHADING", "FEATURE_ROTATE", "FEATURE_IMAGER_CLK_DIVISOR", "FEATURE_TRIG_WITH_CNTRLD_LIGHT", "FEATURE_MAX_PIXEL_SIZE"] ("uFeatureId IN")
            w405 = T20 2 items=["START_STREAM", "PAUSE_STREAM", "STOP_STREAM"] ("uStreamState IN")
            w412 = T22 1 items=["FEATURE_FLAG_PRESENCE                 0x00000001", "FEATURE_FLAG_MANUAL                     0x00000002", "FEATURE_FLAG_AUTO                         0x00000004", "FEATURE_FLAG_ONEPUSH                   0x00000008", "FEATURE_FLAG_OFF                            0x00000010", "FEATURE_FLAG_DESC_SUPPORTED    0x00000020", "FEATURE_FLAG_READ_ONLY               0x00000040"] ("uFlags IN")
            w399 = T21 22 items=["FEATURE_BRIGHTNESS", "FEATURE_EXPOSURE", "FEATURE_SHARPNESS", "FEATURE_WHITE_BAL", "FEATURE_HUE", "FEATURE_SATURATION", "FEATURE_GAMMA", "FEATURE_SHUTTER", "FEATURE_GAIN", "FEATURE_IRIS", "FEATURE_FOCUS", "FEATURE_TEMPERATURE", "FEATURE_TRIGGER", "FEATURE_ZOOM", "FEATURE_PAN", "FEATURE_TILT", "FEATURE_OPT_FILTER", "FEATURE_GPIO", "FEATURE_FRAME_RATE", "FEATURE_ROI", "FEATURE_FLIP", "FEATURE_PIXEL_ADDRESSING", "FEATURE_PIXEL_FORMAT", "FEATURE_EXTENDED_SHUTTER", "FEATURE_AUTO_ROI", "FEATURE_LOOKUP_TABLE", "FEATURE_MEMORY_CHANNEL", "FEATURE_WHITE_SHADING", "FEATURE_ROTATE", "FEATURE_IMAGER_CLK_DIVISOR", "FEATURE_TRIG_WITH_CNTRLD_LIGHT", "FEATURE_MAX_PIXEL_SIZE"] ("uFeatureId IN")
            n116 = event-data() -> ("NewVal"=w390:T3)  [unwired: 1 in, 4 out]
            n117 = To Double Precision Float(number=w390) -> (double precision float=w410:dbl)
            n118 = call <vilib>:"MEPU-Acquisition-SetStreamState.vi"("hCamera IN"=w409, "uStreamState IN"=w405, "Error IN"=w408) -> ("hCamera OUT"=w407:u32, "Error OUT"=w406:errorcluster)  [unwired: 11 in]
            n119 = Build Array(w410) -> (w411:dbl[])
            n120 = call <vilib>:"MEPU-CameraFeatures-SetFeature.vi"("hCamera IN"=w407, "uFeatureId IN"=w399, "uFlags IN"=w412, "pParms IN"=w411, "Error IN"=w406) -> ("hCamera OUT"=w396:u32, "Error OUT"=w392:errorcluster)  [unwired: 8 in, 1 out]
            n121 = case shown="Error" w392 {
              tunnel: [w423 errorcluster {"status"=FALSE, "code"=0, "source"=""} ("Error OUT")] -> w391
              tunnel: w392 -> [w423 _]
              frame No Error {
              }
              frame Error {
                n122 = One Button Dialog(message="Ocurrio un error con el tipo de formato") -> ()  [unwired: 1 in, 1 out]
              }
            }
            n123 = call <vilib>:"MEPU-CameraFeatures-GetFeature.vi"("hCamera IN"=w396, "uFeatureId IN"=w394, "Error IN"=w391) -> ("hCamera OUT"=w395:u32, "pParms OUT"=w393:dbl[], "Error OUT"=w397:errorcluster)  [unwired: 8 in, 2 out]
            n124 = Index Array(array=w393, index=0) -> (element=w388:dbl)
            n125 = property on="Pixel Format Requerido" class="Ring (strict)"("Value"=w388) -> ()  [unwired: 2 in, 2 out]
            n126 = case shown="True" w401 {
              tunnel: w395 -> [w416 w421]
              tunnel: w397 -> [w415 w420]
              tunnel: [w413 w419] -> w402
              tunnel: [w414 w418] -> w403
              frame False {
                w417 = T20 2 items=["START_STREAM", "PAUSE_STREAM", "STOP_STREAM"] ("uStreamState IN")
                n127 = call <vilib>:"MEPU-Acquisition-SetStreamState.vi"("hCamera IN"=w416, "uStreamState IN"=w417, "Error IN"=w415) -> ("hCamera OUT"=w414:u32, "Error OUT"=w413:errorcluster)  [unwired: 11 in]
              }
              frame True {
                w422 = T20 0 items=["START_STREAM", "PAUSE_STREAM", "STOP_STREAM"] ("uStreamState IN")
                n128 = call <vilib>:"MEPU-Acquisition-SetStreamState.vi"("hCamera IN"=w421, "uStreamState IN"=w422, "Error IN"=w420) -> ("hCamera OUT"=w418:u32, "Error OUT"=w419:errorcluster)  [unwired: 11 in]
              }
            }
          }
          event "Exposure Time (ms)": Value Change {
            w448 = T21 7 items=["FEATURE_BRIGHTNESS", "FEATURE_EXPOSURE", "FEATURE_SHARPNESS", "FEATURE_WHITE_BAL", "FEATURE_HUE", "FEATURE_SATURATION", "FEATURE_GAMMA", "FEATURE_SHUTTER", "FEATURE_GAIN", "FEATURE_IRIS", "FEATURE_FOCUS", "FEATURE_TEMPERATURE", "FEATURE_TRIGGER", "FEATURE_ZOOM", "FEATURE_PAN", "FEATURE_TILT", "FEATURE_OPT_FILTER", "FEATURE_GPIO", "FEATURE_FRAME_RATE", "FEATURE_ROI", "FEATURE_FLIP", "FEATURE_PIXEL_ADDRESSING", "FEATURE_PIXEL_FORMAT", "FEATURE_EXTENDED_SHUTTER", "FEATURE_AUTO_ROI", "FEATURE_LOOKUP_TABLE", "FEATURE_MEMORY_CHANNEL", "FEATURE_WHITE_SHADING", "FEATURE_ROTATE", "FEATURE_IMAGER_CLK_DIVISOR", "FEATURE_TRIG_WITH_CNTRLD_LIGHT", "FEATURE_MAX_PIXEL_SIZE"] ("uFeatureId IN")
            w462 = T20 2 items=["START_STREAM", "PAUSE_STREAM", "STOP_STREAM"] ("uStreamState IN")
            w468 = T22 1 items=["FEATURE_FLAG_PRESENCE                 0x00000001", "FEATURE_FLAG_MANUAL                     0x00000002", "FEATURE_FLAG_AUTO                         0x00000004", "FEATURE_FLAG_ONEPUSH                   0x00000008", "FEATURE_FLAG_OFF                            0x00000010", "FEATURE_FLAG_DESC_SUPPORTED    0x00000020", "FEATURE_FLAG_READ_ONLY               0x00000040"] ("uFlags IN")
            w469 = T21 7 items=["FEATURE_BRIGHTNESS", "FEATURE_EXPOSURE", "FEATURE_SHARPNESS", "FEATURE_WHITE_BAL", "FEATURE_HUE", "FEATURE_SATURATION", "FEATURE_GAMMA", "FEATURE_SHUTTER", "FEATURE_GAIN", "FEATURE_IRIS", "FEATURE_FOCUS", "FEATURE_TEMPERATURE", "FEATURE_TRIGGER", "FEATURE_ZOOM", "FEATURE_PAN", "FEATURE_TILT", "FEATURE_OPT_FILTER", "FEATURE_GPIO", "FEATURE_FRAME_RATE", "FEATURE_ROI", "FEATURE_FLIP", "FEATURE_PIXEL_ADDRESSING", "FEATURE_PIXEL_FORMAT", "FEATURE_EXTENDED_SHUTTER", "FEATURE_AUTO_ROI", "FEATURE_LOOKUP_TABLE", "FEATURE_MEMORY_CHANNEL", "FEATURE_WHITE_SHADING", "FEATURE_ROTATE", "FEATURE_IMAGER_CLK_DIVISOR", "FEATURE_TRIG_WITH_CNTRLD_LIGHT", "FEATURE_MAX_PIXEL_SIZE"] ("uFeatureId IN")
            n129 = event-data() -> ("NewVal"=w443:dbl)  [unwired: 1 in, 4 out]
            n130 = Divide(x=w443, y=1000.0) -> (x/y=w455:dbl)
            n131 = call <vilib>:"MEPU-Acquisition-SetStreamState.vi"("hCamera IN"=w458, "uStreamState IN"=w462, "Error IN"=w457) -> ("hCamera OUT"=w464:u32, "Error OUT"=w463:errorcluster)  [unwired: 11 in]
            n132 = To Double Precision Float(number=w455) -> (double precision float=w466:dbl)
            n133 = Build Array(w466) -> (w467:dbl[])
            n134 = call <vilib>:"MEPU-CameraFeatures-SetFeature.vi"("hCamera IN"=w464, "uFeatureId IN"=w469, "uFlags IN"=w468, "pParms IN"=w467, "Error IN"=w463) -> ("hCamera OUT"=w447:u32, "Error OUT"=w465:errorcluster)  [unwired: 8 in, 1 out]
            n135 = case shown="No Error" w465 {
              tunnel: [w480 errorcluster {"status"=FALSE, "code"=0, "source"=""} ("Error OUT")] -> w444
              tunnel: w465 -> [w480 _]
              frame No Error {
              }
              frame Error {
                n136 = One Button Dialog(message="Ocurrio un error con shutter time") -> ()  [unwired: 1 in, 1 out]
              }
            }
            n137 = call <vilib>:"MEPU-CameraFeatures-GetFeature.vi"("hCamera IN"=w447, "uFeatureId IN"=w448, "Error IN"=w444) -> ("hCamera OUT"=w446:u32, "pParms OUT"=w449:dbl[], "Error OUT"=w445:errorcluster)  [unwired: 8 in, 2 out]
            n138 = Unbundle By Name(w429) -> ("Minimum Value"=w433:dbl, "Maximum Value"=w432:dbl, "Physical Channel"=w431:tag, "DAQ Fs (S/s)"=w430:dbl)
            n139 = Index Array(array=w449, index=0) -> (element=w452:dbl)
            n140 = case shown="True" w456 {
              tunnel: w445 -> [w473 w478]
              tunnel: [w471 w477] -> w459
              tunnel: [w472 w476] -> w460
              tunnel: w446 -> [w470 w475]
              frame False {
                w474 = T20 2 items=["START_STREAM", "PAUSE_STREAM", "STOP_STREAM"] ("uStreamState IN")
                n141 = call <vilib>:"MEPU-Acquisition-SetStreamState.vi"("hCamera IN"=w470, "uStreamState IN"=w474, "Error IN"=w473) -> ("hCamera OUT"=w472:u32, "Error OUT"=w471:errorcluster)  [unwired: 11 in]
              }
              frame True {
                w479 = T20 0 items=["START_STREAM", "PAUSE_STREAM", "STOP_STREAM"] ("uStreamState IN")
                n142 = call <vilib>:"MEPU-Acquisition-SetStreamState.vi"("hCamera IN"=w475, "uStreamState IN"=w479, "Error IN"=w478) -> ("hCamera OUT"=w476:u32, "Error OUT"=w477:errorcluster)  [unwired: 11 in]
              }
            }
            n143 = Multiply(x=w452, y=1000) -> (x*y=w435:dbl)
            n144 = property on="Exposure Time (ms)" class="Slide (strict)"("Value"=w435) -> ()  [unwired: 2 in, 2 out]
            n145 = Divide(x=w435, y=sgl 1000.0) -> (x/y=w436:dbl)
            n146 = call "Restart DAQ.vi"("Min Value"=w433, "tiempo (s)"=w436, "Max Value"=w432, "error IN"=w437, "Fs (S/s)"=w430, "Physical Channel"=w431, "task IN"=w438) -> ("error OUT"=w440:errorcluster, "# samples"=w439:u32, "task OUT"=w434:refnum<k21>)  [unwired: 2 in]
          }
          event "DAQ Parameters": Value Change {
            n147 = event-data() -> ("NewVal"=w487:T4)  [unwired: 1 in, 4 out]
            n148 = Unbundle By Name(w487) -> ("Minimum Value"=w486:dbl, "Maximum Value"=w483:dbl, "Physical Channel"=w485:tag, "DAQ Fs (S/s)"=w484:dbl)
            n149 = call "Restart DAQ.vi"("Min Value"=w486, "tiempo (s)"=w493, "Max Value"=w483, "error IN"=w495, "Fs (S/s)"=w484, "Physical Channel"=w485, "task IN"=w496) -> ("error OUT"=w492:errorcluster, "# samples"=w491:u32, "task OUT"=w494:refnum<k21>)  [unwired: 2 in]
          }
          event "Gain": Value Change {
            w516 = T21 8 items=["FEATURE_BRIGHTNESS", "FEATURE_EXPOSURE", "FEATURE_SHARPNESS", "FEATURE_WHITE_BAL", "FEATURE_HUE", "FEATURE_SATURATION", "FEATURE_GAMMA", "FEATURE_SHUTTER", "FEATURE_GAIN", "FEATURE_IRIS", "FEATURE_FOCUS", "FEATURE_TEMPERATURE", "FEATURE_TRIGGER", "FEATURE_ZOOM", "FEATURE_PAN", "FEATURE_TILT", "FEATURE_OPT_FILTER", "FEATURE_GPIO", "FEATURE_FRAME_RATE", "FEATURE_ROI", "FEATURE_FLIP", "FEATURE_PIXEL_ADDRESSING", "FEATURE_PIXEL_FORMAT", "FEATURE_EXTENDED_SHUTTER", "FEATURE_AUTO_ROI", "FEATURE_LOOKUP_TABLE", "FEATURE_MEMORY_CHANNEL", "FEATURE_WHITE_SHADING", "FEATURE_ROTATE", "FEATURE_IMAGER_CLK_DIVISOR", "FEATURE_TRIG_WITH_CNTRLD_LIGHT", "FEATURE_MAX_PIXEL_SIZE"] ("uFeatureId IN")
            w526 = T20 2 items=["START_STREAM", "PAUSE_STREAM", "STOP_STREAM"] ("uStreamState IN")
            w532 = T22 1 items=["FEATURE_FLAG_PRESENCE                 0x00000001", "FEATURE_FLAG_MANUAL                     0x00000002", "FEATURE_FLAG_AUTO                         0x00000004", "FEATURE_FLAG_ONEPUSH                   0x00000008", "FEATURE_FLAG_OFF                            0x00000010", "FEATURE_FLAG_DESC_SUPPORTED    0x00000020", "FEATURE_FLAG_READ_ONLY               0x00000040"] ("uFlags IN")
            w533 = T21 8 items=["FEATURE_BRIGHTNESS", "FEATURE_EXPOSURE", "FEATURE_SHARPNESS", "FEATURE_WHITE_BAL", "FEATURE_HUE", "FEATURE_SATURATION", "FEATURE_GAMMA", "FEATURE_SHUTTER", "FEATURE_GAIN", "FEATURE_IRIS", "FEATURE_FOCUS", "FEATURE_TEMPERATURE", "FEATURE_TRIGGER", "FEATURE_ZOOM", "FEATURE_PAN", "FEATURE_TILT", "FEATURE_OPT_FILTER", "FEATURE_GPIO", "FEATURE_FRAME_RATE", "FEATURE_ROI", "FEATURE_FLIP", "FEATURE_PIXEL_ADDRESSING", "FEATURE_PIXEL_FORMAT", "FEATURE_EXTENDED_SHUTTER", "FEATURE_AUTO_ROI", "FEATURE_LOOKUP_TABLE", "FEATURE_MEMORY_CHANNEL", "FEATURE_WHITE_SHADING", "FEATURE_ROTATE", "FEATURE_IMAGER_CLK_DIVISOR", "FEATURE_TRIG_WITH_CNTRLD_LIGHT", "FEATURE_MAX_PIXEL_SIZE"] ("uFeatureId IN")
            n150 = event-data() -> ("NewVal"=w510:dbl)  [unwired: 1 in, 4 out]
            n151 = To Double Precision Float(number=w510) -> (double precision float=w530:dbl)
            n152 = call <vilib>:"MEPU-Acquisition-SetStreamState.vi"("hCamera IN"=w522, "uStreamState IN"=w526, "Error IN"=w521) -> ("hCamera OUT"=w528:u32, "Error OUT"=w527:errorcluster)  [unwired: 11 in]
            n153 = Build Array(w530) -> (w531:dbl[])
            n154 = call <vilib>:"MEPU-CameraFeatures-SetFeature.vi"("hCamera IN"=w528, "uFeatureId IN"=w533, "uFlags IN"=w532, "pParms IN"=w531, "Error IN"=w527) -> ("hCamera OUT"=w515:u32, "Error OUT"=w529:errorcluster)  [unwired: 8 in, 1 out]
            n155 = case shown="Error" w529 {
              tunnel: [w544 errorcluster {"status"=FALSE, "code"=0, "source"=""} ("Error OUT")] -> w512
              tunnel: w529 -> [w544 _]
              frame No Error {
              }
              frame Error {
                n156 = One Button Dialog(message="Ocurrio un error con Gain") -> ()  [unwired: 1 in, 1 out]
              }
            }
            n157 = call <vilib>:"MEPU-CameraFeatures-GetFeature.vi"("hCamera IN"=w515, "uFeatureId IN"=w516, "Error IN"=w512) -> ("hCamera OUT"=w514:u32, "pParms OUT"=w517:dbl[], "Error OUT"=w513:errorcluster)  [unwired: 8 in, 2 out]
            n158 = case shown="True" w520 {
              tunnel: w513 -> [w537 w542]
              tunnel: [w535 w541] -> w523
              tunnel: [w536 w540] -> w524
              tunnel: w514 -> [w534 w539]
              frame False {
                w538 = T20 2 items=["START_STREAM", "PAUSE_STREAM", "STOP_STREAM"] ("uStreamState IN")
                n159 = call <vilib>:"MEPU-Acquisition-SetStreamState.vi"("hCamera IN"=w534, "uStreamState IN"=w538, "Error IN"=w537) -> ("hCamera OUT"=w536:u32, "Error OUT"=w535:errorcluster)  [unwired: 11 in]
              }
              frame True {
                w543 = T20 0 items=["START_STREAM", "PAUSE_STREAM", "STOP_STREAM"] ("uStreamState IN")
                n160 = call <vilib>:"MEPU-Acquisition-SetStreamState.vi"("hCamera IN"=w539, "uStreamState IN"=w543, "Error IN"=w542) -> ("hCamera OUT"=w540:u32, "Error OUT"=w541:errorcluster)  [unwired: 11 in]
              }
            }
            n161 = Index Array(array=w517, index=0) -> (element=w509:dbl)
            n162 = property on="Gain" class="Slide (strict)"("Value"=w509) -> ()  [unwired: 2 in, 2 out]
          }
        }
        n163 = Tick Count (ms)() -> (millisecond timer value=w76:u32)
        n164 = Subtract(x=w76, y=w77) -> (x-y=→"time elapsed (ms)":u32)
        n165 = call <vilib>:"Simple Error Handler.vi"("error in (no error)"=w126) -> ("error out"=w130:errorcluster)  [unwired: 1 in, 7 out]
        n166 = case shown="Error" w130 {
          selector: w130 -> [w136 _]
          tunnel: [w136 errorcluster {"status"=FALSE, "code"=0, "source"=""} ("error IO")] -> w106
          tunnel: [FALSE ("T button?") w138] -> w129
          frame No Error {
          }
          frame Error {
            n167 = Two Button Dialog(message="An error was detected.\nDo you wish to continue execution?", 1:"Stop" ("F button name (\"Cancel\")"), 2:"Continue" ("T button name (\"OK\")")) -> (T button?=w139:bool)
            n168 = Not(x=w139) -> (.not. x?=w138:bool)
          }
        }
        n169 = call "todo.vi"("error IO 2"=w123) -> ("error IO"=w113:errorcluster, "T button?"=w120:bool)
        n170 = property on="Stop App" class="Bool (strict)"() -> ("Value"=w122:bool)  [unwired: 2 in, 2 out]
        n171 = property on="Stop App" class="Bool (strict)"() -> ("Value"=w127:bool)  [unwired: 2 in, 2 out]
        n172 = Or(x=w120, y=w122) -> (x .or. y?=w110:bool)
        n173 = Or(x=w129, y=w127) -> (x .or. y?=w111:bool)
        n174 = Or(x=w111, y=w110) -> (x .or. y?=w121:bool)
      }
      n175 = call <vilib>:"MEPU-Initialization-Uninitialize.vi"("hCamera IN"=w70, "Error IN"=w54) -> ("Error OUT"=w22:errorcluster)  [unwired: 13 in]
      n176 = call <vilib>:"DAQmx Clear Task.vi"("task in"=w37, "error in"=w36) -> ("error out"=w39:errorcluster)  [unwired: 13 in]
      n177 = call <vilib>:"Sound Output Clear.vi"("error in (no error)"=w26, "task ID"=w27) -> ("error out"=w24:errorcluster)  [unwired: 9 in]
      n178 = call <vilib>:"Simple Error Handler.vi"("type of dialog (OK msg:1)"=w38, "error in (no error)"=w39) -> ()  [unwired: 3 in, 5 out]
      n179 = call <vilib>:"Simple Error Handler.vi"("type of dialog (OK msg:1)"=w23, "error in (no error)"=w22) -> ()  [unwired: 3 in, 5 out]
      n180 = call <vilib>:"Simple Error Handler.vi"("type of dialog (OK msg:1)"=w25, "error in (no error)"=w24) -> ()  [unwired: 3 in, 5 out]
    }
  }
